vi "Initialize.vi"(7 "VI Ref":variant, 8 "error in (no error)":errorcluster, 9 "Wizard Interface":T1, 10 "MetaDataObj in":refnum<class "MetaDataObj.lvclass">, 11 "ConfirmQuitSpecPage in":refnum<class "ConfirmQuitSpecPage.lvclass">) -> (0 "error out":errorcluster, 3 "ConfirmQuitSpecPage out":refnum<class "ConfirmQuitSpecPage.lvclass">)   [LabVIEW 2016, in "ConfirmQuitSpecPage.lvclass"]
uses:
  <resource>/dialog/NewProjectWizard/SpecPage/ConfirmQuitSpecPage/ConfirmQuitSpecPage.lvclass
  <resource>/dialog/NewProjectWizard/MetaDataObj/MetaDataObj.lvclass
  <resource>/dialog/NewProjectWizard/Spec Page Interface.ctl
  <resource>/dialog/NewProjectWizard/Spec Page Interface Confirm Quit.ctl
  <resource>/dialog/NewProjectWizard/SpecPage/ConfirmQuitSpecPage/ConfirmQuitSpecPage.lvclass/ConfirmQuitSpecPage.ctl
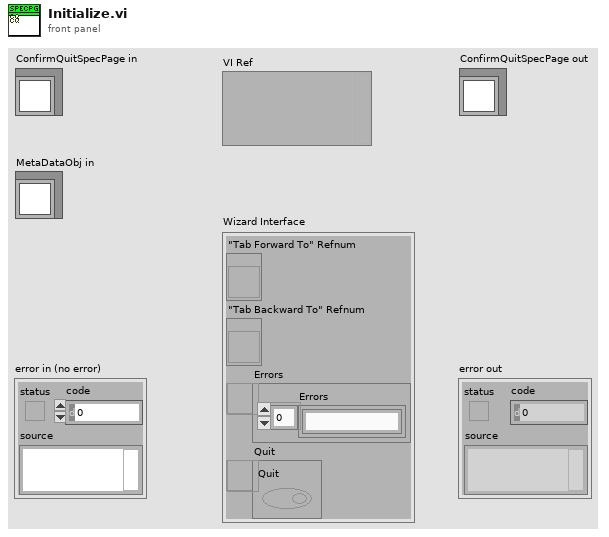
[diagram p1: front panel]
types:
  T1 = typedef "Spec Page Interface.ctl" = cluster{"\"Tab Forward To\" Refnum":refnum<vi>, "\"Tab Backward To\" Refnum":refnum<vi>, "Errors":refnum<user-event>, "Quit":refnum<user-event>}
  T2 = typedef "Spec Page Interface Confirm Quit.ctl" = cluster{"\"Tab Forward To\" Refnum":refnum<vi>, "\"Tab Backward To\" Refnum":refnum<vi>, "Errors":refnum<user-event>, "Quit":refnum<user-event>, "Additional Data":variant}
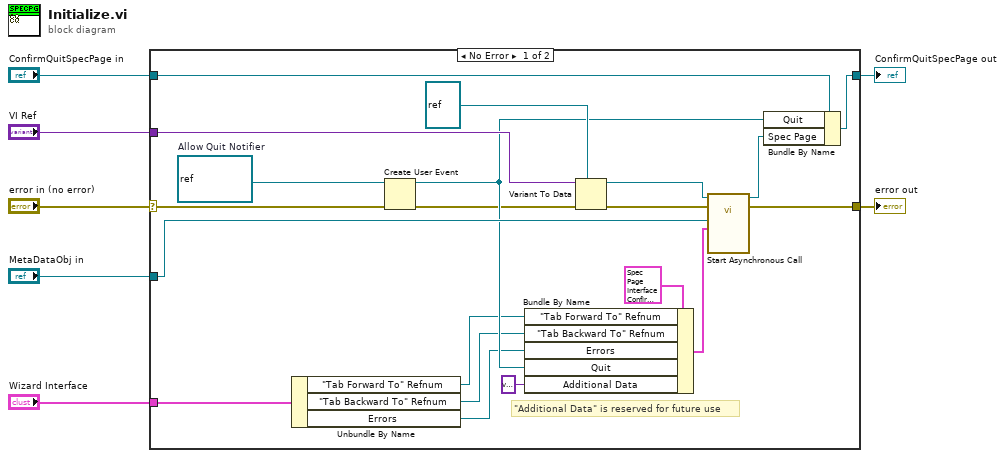
[diagram p0: block diagram]
diagram:
  n1 = case shown="No Error" "error in (no error)" {
    selector: "error in (no error)" -> [w12 w28]
    tunnel: "VI Ref" -> [w27 _]
    tunnel: "MetaDataObj in" -> [w22 _]
    tunnel: "ConfirmQuitSpecPage in" -> [w20 w29]
    tunnel: [w19 w29] -> w3
    tunnel: [w11 w28] -> w2
    tunnel: "Wizard Interface" -> [w16 _]
    frame No Error {
      w21 = refnum<notifier> refnum  # Allow Quit Notifier
      # "\"Additional Data\" is reserved for future use"
      n2 = Unbundle By Name(w16) -> ("\"Tab Forward To\" Refnum"=w15:refnum<vi>, "\"Tab Backward To\" Refnum"=w14:refnum<vi>, "Errors"=w13:refnum<user-event>)
      n3 = Create User Event(user event datatype=w21, error in=w12) -> (user event=w18:refnum<user-event>, error out=w10:errorcluster)
      n4 = Bundle By Name(cluster=T2 {"\"Tab Forward To\" Refnum"=refnum, "\"Tab Backward To\" Refnum"=refnum, "Errors"=refnum, "Quit"=refnum, "Additional Data"=variant} ("Spec Page Interface"), "\"Tab Forward To\" Refnum"=w15, "\"Tab Backward To\" Refnum"=w14, "Errors"=w13, "Quit"=w18, "Additional Data"=variant) -> (w23:T2)
      n5 = Variant To Data(error in=w10, type=refnum<vi> refnum ("reference"), Variant=w27) -> (data=w25:refnum<vi>, error out=w9:errorcluster)
      n6 = call-by-ref "Start Asynchronous Call"(reference=w25, error in=w9, "Spec Page Interface"=w23, "MetaDataObj in"=w22) -> (reference out=w17:refnum<vi>, error out=w11:errorcluster)  [unwired: 9 in, 1 out]
      n7 = Bundle By Name(cluster=w20, "Quit"=w18, "Spec Page"=w17) -> (w19:refnum<class "ConfirmQuitSpecPage.lvclass">)
    }
    frame Error {
    }
  }
  "error out" <- w2
  "ConfirmQuitSpecPage out" <- w3
